vi "Test_MergeErrorsPublication_WarningCluster_WarningIgnored.vi"(8 "error in (no error)":errorcluster, 11 "TestCase in":refnum<class "TestPublicationPolicy.lvclass">) -> (0 "error out":errorcluster, 3 "TestCase out":refnum<class "TestPublicationPolicy.lvclass">)   [LabVIEW 2017, in "TestPublicationPolicy.lvclass"]
uses:
  TestPublicationPolicy.lvclass
  gpm_packages/@cs/mva-core/Source/IMediator/MutexedPublishRequest/MutexedPublishRequest.lvclass
  gpm_packages/@cs/mva-core/Source/IMediator/IPublicationPolicy/IPublicationPolicy.lvclass
  gpm_packages/@cs/mva-core/Source/PublicationPolicy/MergeErrorsPublication/MergeErrorsPublication.lvclass
  gpm_packages/@cs/transport/Source/Concrete/NotifierTransport/NotifierTransport.lvclass
  C:/Git/mva-framework/Source/Framework/IMediator/IPublicationPolicy/IPublicationPolicy.lvclass
  C:/Git/mva-framework/gpm_packages/@cs/transport/Source/ITransport/ITransport.lvclass
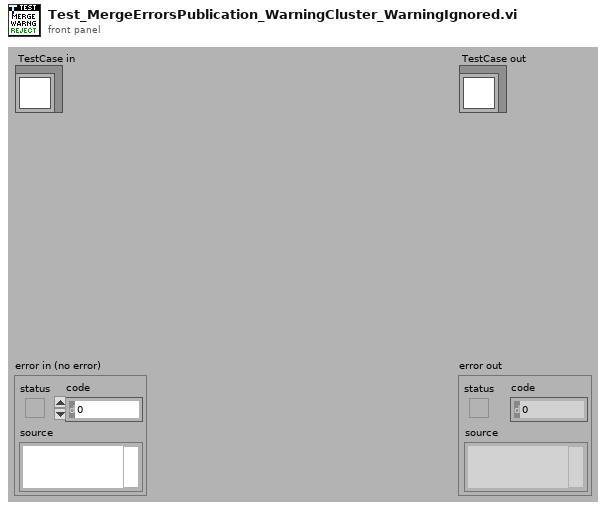
[diagram p1: front panel]
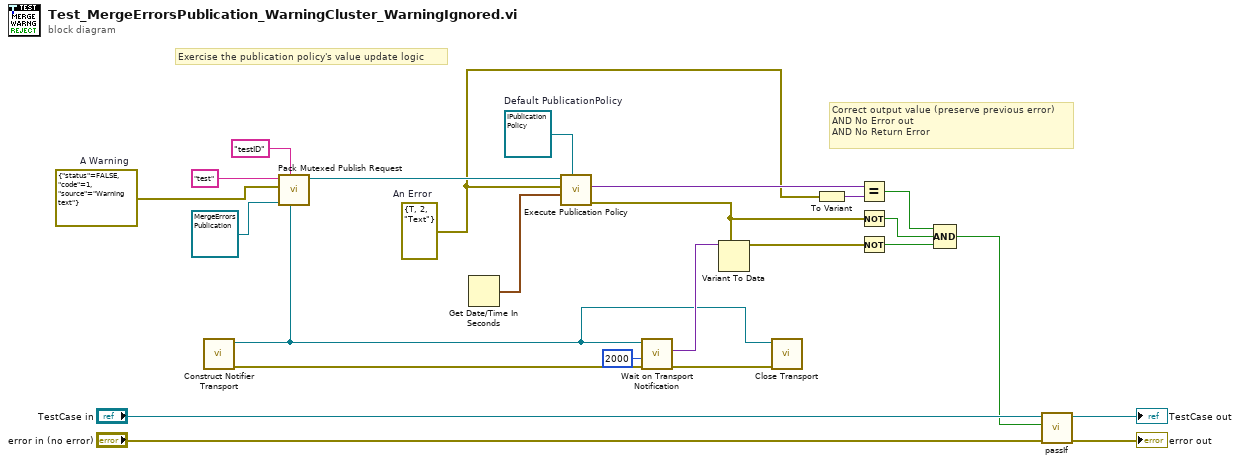
[diagram p0: block diagram]
diagram:
  w5 = errorcluster {"status"=FALSE, "code"=1, "source"="Warning text"}  # A Warning
  w18 = refnum<class "IPublicationPolicy.lvclass"> refnum  # Default PublicationPolicy
  w3 = errorcluster {"status"=TRUE, "code"=2, "source"="Text"}  # An Error
  # "Correct output value (preserve previous error)\nAND No Error out\nAND No Return Error"
  # "Exercise the publication policy's value update logic"
  n1 = call "Construct Notifier Transport.vi"() -> ("error out"=w15:errorcluster, "NotifierTransport"=w2:refnum<class "NotifierTransport.lvclass">)  [unwired: 10 in]
  n2 = call "Pack Mutexed Publish Request.vi"("Return Error Transport"=w2, "Publisher ID"="testID", "error in (no error)"=refnum<class "MergeErrorsPublication.lvclass"> refnum ("PublicationPolicy.lvlib:MergeErrorsPublication.lvclass"), "Datum Value or Type"=w5, "Datum Name"="test") -> ("MutexedPublishRequest Out"=w20:refnum<class "MutexedPublishRequest.lvclass">)  [unwired: 5 in, 1 out]
  n3 = Get Date/Time In Seconds() -> (seconds since 1Jan1904=w21:timestamp)
  n4 = call-dynamic "Execute Publication Policy.vi"("Default PublicationPolicy"=w18, "Last Publish Time"=w21, "Last Published Value"=w3, "MutexedPublishRequest"=w20) -> ("error out (Reject Publication)"=w7:errorcluster, "Value to Publish"=w12:variant)  [unwired: 5 in, 1 out]
  n5 = call "Wait on Transport Notification.vi"("error in (no error)"=w15, "Timeout In ms (-1)"=2000, "NotifierTransport"=w2) -> ("error out"=w1:errorcluster, "Data"=w13:variant)  [unwired: 6 in, 1 out]
  n6 = Variant To Data(type=w7, Variant=w13) -> (data=w10:errorcluster)  [unwired: 1 in, 1 out]
  n7 = call-dynamic "Close Transport.vi"("error in (no error)"=w1, "NotifierTransport"=w2) -> ()  [unwired: 9 in, 1 out]
  n8 = To Variant(anything=w3) -> (Variant=w11:variant)
  n9 = Equal?(x=w12, y=w11) -> (x = y?=w9:bool)
  n10 = Not(x=w7) -> (.not. x?=w6:bool)
  n11 = Not(x=w10) -> (.not. x?=w8:bool)
  n12 = Compound Arithmetic op=AND(w9, w6, w8) -> (w4:bool)
  n13 = call-dynamic "passIf.vi"("error in (no error)"="error in (no error)", "pass"=w4, "TestCase in"="TestCase in") -> ("error out"=→"error out":errorcluster, "TestCase out"=→"TestCase out":refnum<class "TestPublicationPolicy.lvclass">)  [unwired: 7 in]
